vi "SanityPressureCull.vi"(10 "GoodPressures":T1, 11 "VmagUVWCone":dbl[][](array[numeric])) -> (2 "SanitisedVmagUVWCone":dbl[][](array[numeric]))   [LabVIEW 2013]
uses:
  GoodArray.ctl
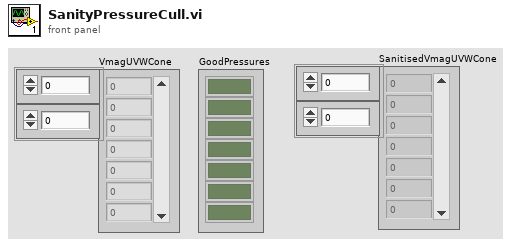
[diagram p1: front panel]
types:
  T1 = typedef "GoodArray.ctl" = bool[]
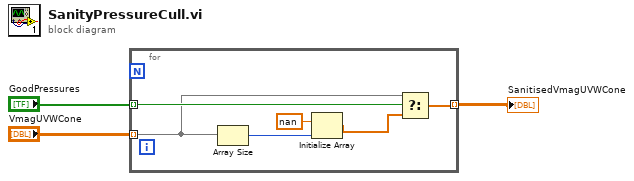
[diagram p0: block diagram]
diagram:
  n1 = for {
    tunnel: [w9] -> w2 mode=indexing
    tunnel: "VmagUVWCone" -> [w4] mode=indexing
    tunnel: "GoodPressures" -> [w6] mode=indexing
    n2 = Array Size(array=w4) -> (size(s)=w8:i32)
    n3 = Initialize Array(nan ("element"), w8) -> (w5:dbl[])
    n4 = Select(t=w4, s=w6, f=w5) -> (s? t:f=w9:dbl[])
  }
  "SanitisedVmagUVWCone" <- w2
